vi "array_diff.vi"(4 "array in":i32[](array[numeric])=[-5, 7]) -> (1 "arrout out":i32[](array[numeric]))   [LabVIEW 2015]
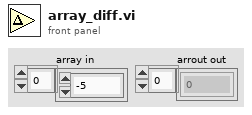
[diagram p1: front panel]
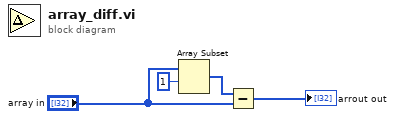
[diagram p0: block diagram]
diagram:
  n1 = Array Subset(array="array in", index=1) -> (w3:i32[])  [unwired: 1 in]
  n2 = Subtract(x=w3, y="array in") -> (x-y=→"arrout out":i32[])
